vi "CFindSCU.vi"() -> ()   [LabVIEW 2013]
panel:
  in  "query model":string=" -P "
  out "command":string
  in  "DicomFile":string
  out "return code":i32
  in  "port":string="11112"
  in  "server(ip)":string="www.dicomserver.co.uk "
  in  "aec":string="ANY-SCP"
  in  "aet":string="SCU"
  in  "standard input":string="-v -aet SCU -aec ANY-SCP www.dicomserver.co.uk 11112"
  in  "executable path":string="../DICOM/dcmtk/bin/echoscu.exe"
  in  "error in (no error)":errorcluster
  out "error out":errorcluster
  out "standard error":string
  out "standard output":string
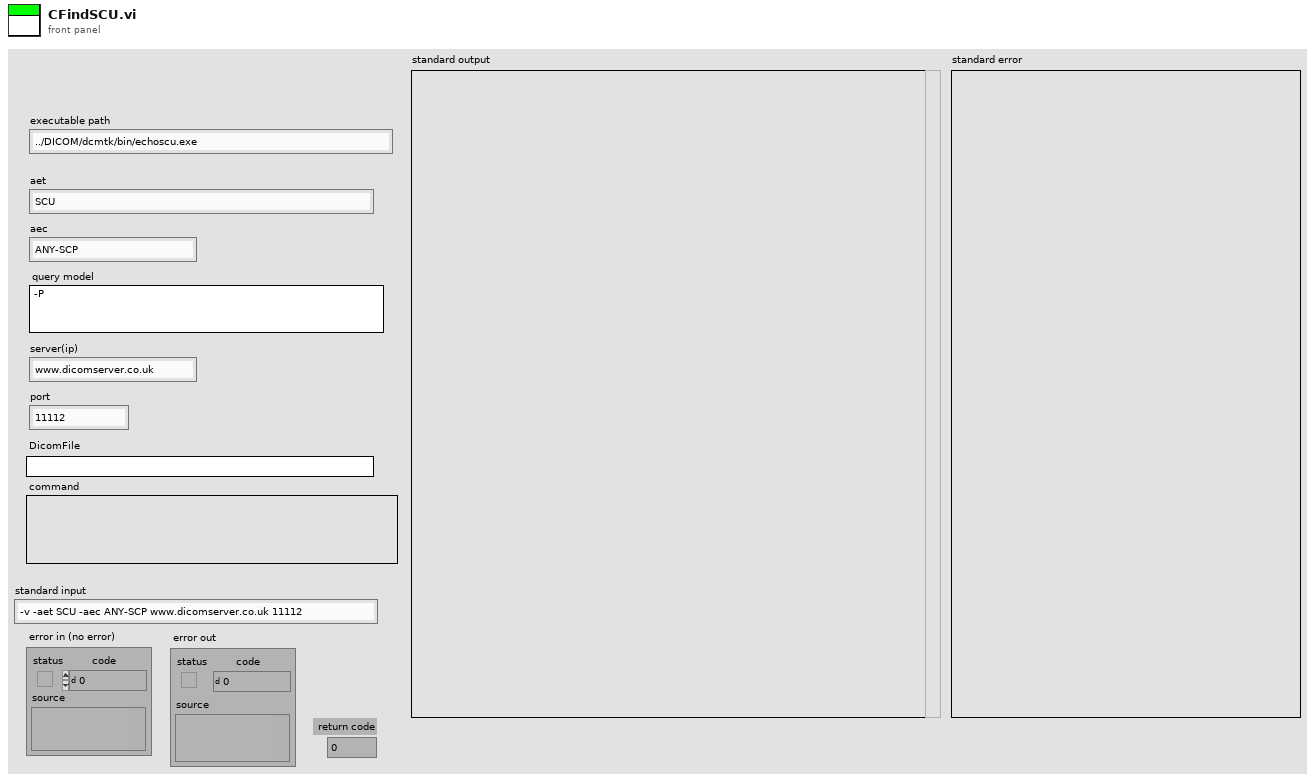
[diagram p1: front panel]
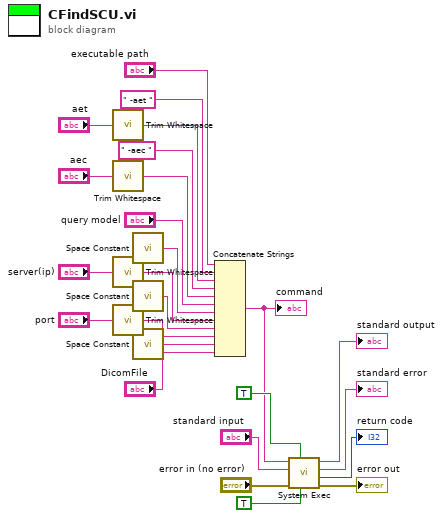
[diagram p0: block diagram]
diagram:
  n1 = call <vilib>:"Trim Whitespace.vi"("string"="aet") -> ("trimmed string"=w13:string)  [unwired: 1 in]
  n2 = call <vilib>:"Trim Whitespace.vi"("string"="aec") -> ("trimmed string"=w11:string)  [unwired: 1 in]
  n3 = call <vilib>:"Trim Whitespace.vi"("string"="server(ip)") -> ("trimmed string"=w3:string)  [unwired: 1 in]
  n4 = call <vilib>:"Trim Whitespace.vi"("string"="port") -> ("trimmed string"=w8:string)  [unwired: 1 in]
  n5 = call <vilib>:"Space Constant.vi"() -> ("String"=w2:string)
  n6 = call <vilib>:"Space Constant.vi"() -> ("String"=w10:string)
  n7 = call <vilib>:"Space Constant.vi"() -> ("String"=w5:string)
  n8 = Concatenate Strings("executable path", " -aet " ("string"), w13, " -aec " ("string"), w11, "query model", w2, w3, w10, w8, w5, "DicomFile") -> (w18:string)
  "command" <- w18
  n9 = call <vilib>:"System Exec.vi"("run minimized? (F)"=TRUE, "wait until completion? (T)"=TRUE, "error in (no error)"="error in (no error)", "standard input"="standard input", "command line"=w18) -> ("error out"=→"error out":errorcluster, "return code"=→"return code":i32, "standard error"=→"standard error":string, "standard output"=→"standard output":string)  [unwired: 3 in]
